vi "nican_init.vi"() -> (0 "CAN Init":T2)   [LabVIEW 2017]
uses:
  <vilib>/nican/nican.llb/xobjhandle.ctl
  <vilib>/nican/nican.llb/ncNetAttr.ctl
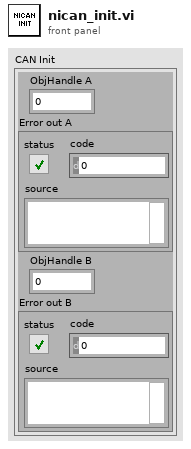
[diagram p1: front panel]
types:
  T1 = typedef "xobjhandle.ctl" = u32
  T2 = cluster{"ObjHandle A":T1, "Error out A":errorcluster, "ObjHandle B":T1, "Error out B":errorcluster}
  T3 = typedef "ncNetAttr.ctl" = cluster{"Start On Open":enum32{"FALSE", "TRUE"}, "Baud Rate":u32, "Read Queue Length":u32, "Write Queue Length":u32, "Standard Comparator":u32, "Standard Mask":u32, "Extended Comparator":u32, "Extended Mask":u32}
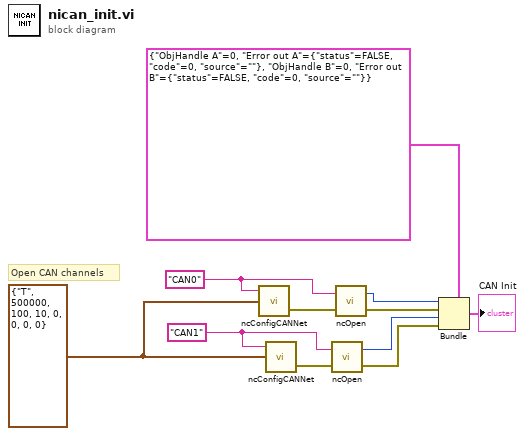
[diagram p0: block diagram]
diagram:
  w10 = "CAN1" ("ObjName")
  w11 = "CAN0" ("ObjName")
  w9 = T3 {"Start On Open"=enum."TRUE", "Baud Rate"=500000, "Read Queue Length"=100, "Write Queue Length"=10, "Standard Comparator"=0, "Standard Mask"=0, "Extended Comparator"=0, "Extended Mask"=0} ("CAN Network Interface Config")
  # "Open CAN channels"
  n1 = call <vilib>:"ncConfigCANNet.vi"("CAN Network Interface Config"=w9, "ObjName"=w11) -> ("Error out"=w8:errorcluster)  [unwired: 3 in]
  n2 = call <vilib>:"ncConfigCANNet.vi"("CAN Network Interface Config"=w9, "ObjName"=w10) -> ("Error out"=w7:errorcluster)  [unwired: 3 in]
  n3 = call <vilib>:"ncOpen.vi"("Error in"=w7, "ObjName"=w10) -> ("Error out"=w2:errorcluster, "ObjHandle out"=w3:T1)
  n4 = call <vilib>:"ncOpen.vi"("Error in"=w8, "ObjName"=w11) -> ("Error out"=w4:errorcluster, "ObjHandle out"=w5:T1)
  n5 = Bundle(cluster=T2 {"ObjHandle A"=0, "Error out A"={"status"=FALSE, "code"=0, "source"=""}, "ObjHandle B"=0, "Error out B"={"status"=FALSE, "code"=0, "source"=""}}, "ObjHandle A"=w5, "Error out A"=w4, "ObjHandle B"=w3, "Error out B"=w2) -> (→"CAN Init":T2)
